vi "FTW-JSON-Lint.vi"(7 "JSON String":string, 11 "error in":errorcluster) -> (8 "Linted JSON":string, 15 "error out":errorcluster)   [LabVIEW 2015]
panel:
  # "Inputs"
  # "Outputs"
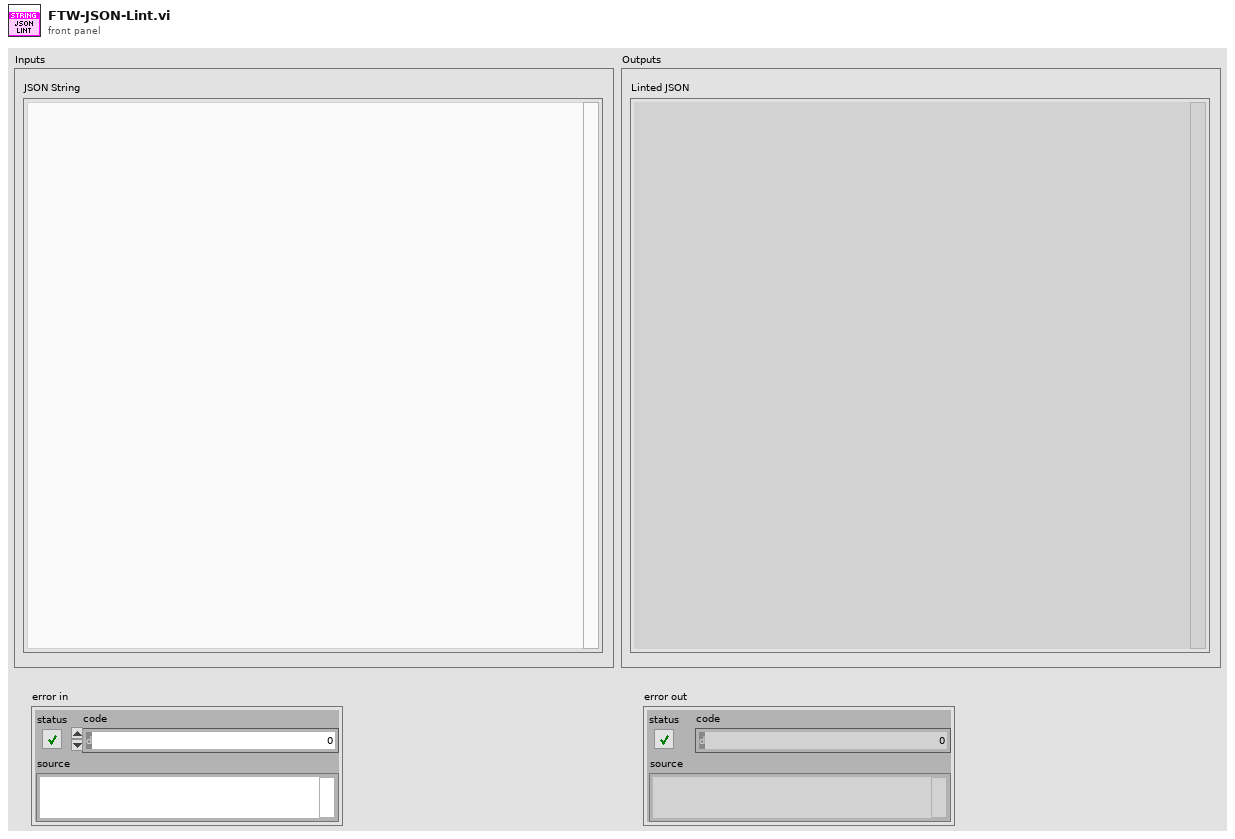
[diagram p1: front panel]
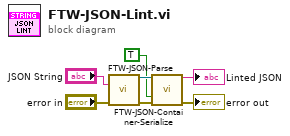
[diagram p0: block diagram]
diagram:
  n1 = call "FTW-JSON-Parse.vi"("JSON String"="JSON String", "error in"="error in") -> ("Container"=w7:refnum<class "FTW-Container.lvclass">, "error out"=w4:errorcluster)  [unwired: 12 in]
  n2 = call "FTW-JSON-Container-Serialize.vi"("Container"=w7, "Pretty Print"=TRUE, "error in"=w4) -> ("JSON String"=→"Linted JSON":string, "error out"=→"error out":errorcluster)  [unwired: 11 in]
